vi "Serial Receive Simulation.vi"() -> ()   [LabVIEW 2013]
uses:
  <vilib>/rvi/DesktopExecutionNode/Execution/niFpgaDEN_Execute.vi
  <vilib>/rvi/DesktopExecutionNode/DesktopExecutionNode.xnode
  Source/I2S-TDM.lvlib
panel:
  out "number":u32
  out "sample bits":bool[](array[boolean])=[TRUE, FALSE, FALSE, FALSE, FALSE, FALSE, FALSE, FALSE, FALSE, FALSE, FALSE, FALSE, FALSE, FALSE, FALSE, FALSE, FALSE, FALSE, FALSE, FALSE, FALSE, FALSE, FALSE, TRUE]
  out "sample":u32
  in  "force stop":bool
  in  "start transfer":bool
  in  "ready for output":bool
  in  "pause":bool
  in  "24-bit data":bool[](array[boolean])=[TRUE, FALSE, FALSE, FALSE, FALSE, FALSE, FALSE, FALSE, FALSE, FALSE, FALSE, FALSE, FALSE, FALSE, FALSE, FALSE, FALSE, FALSE, FALSE, FALSE, FALSE, FALSE, FALSE, TRUE]
  in  "History Size":i32=100
  in  "Reset?":bool
  in  "wait":u32=50
  out "Digital Waveform Graph":digitalwaveform(graph)
  in  "transfer length":u8=32
  in  "stop":bool
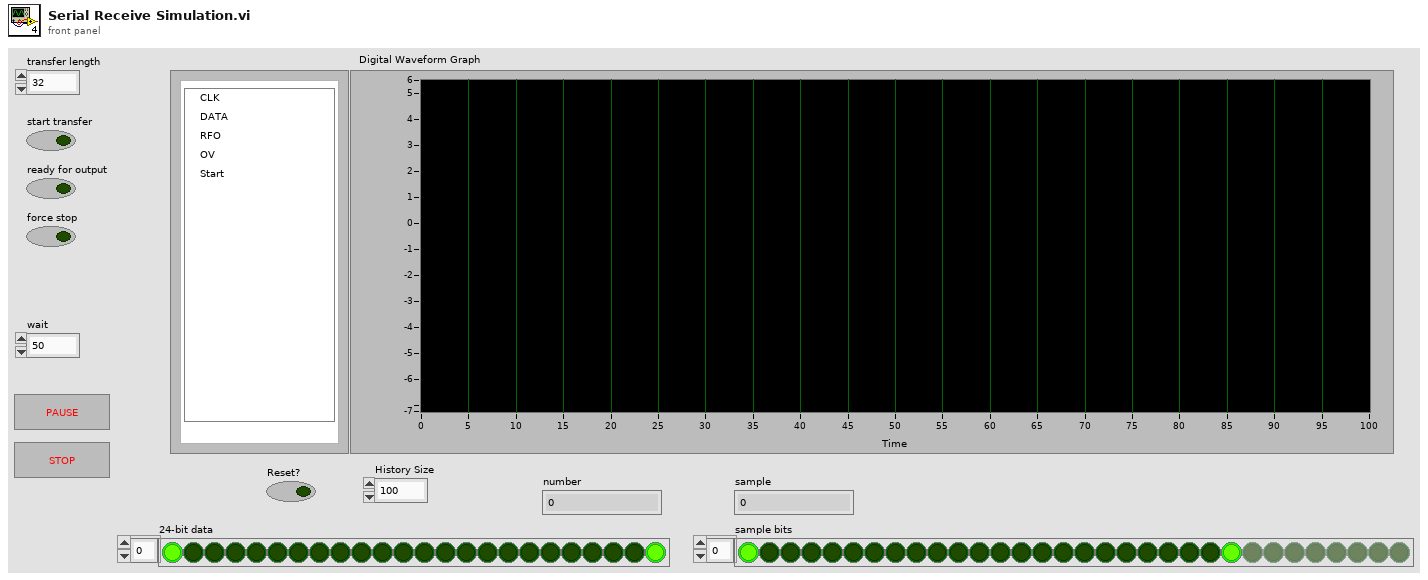
[diagram p1: front panel]
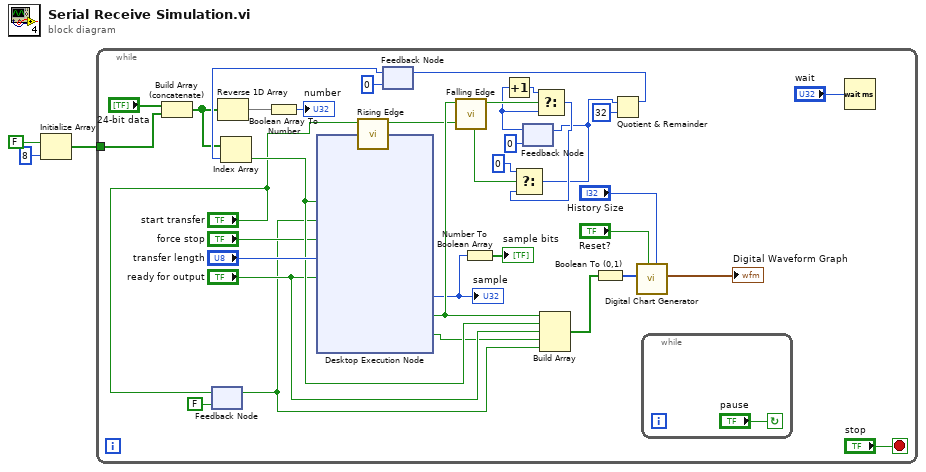
[diagram p0: block diagram]
diagram:
  n1 = Initialize Array(FALSE, 8 ("dimension size")) -> (w1:bool[])
  n2 = while {
    tunnel: w1 -> [w32]
    stop <- "stop" stop-if-true
    n3 = Build Array (concatenate)("24-bit data", w32) -> (w8:bool[])
    n4 = feedback-in #1("start transfer") -> ()
    n5 = feedback #1(FALSE ("start transfer")) -> (w6:bool)
    n6 = Reverse 1D Array(array=w8) -> (reversed array=w4:bool[])
    n7 = Boolean Array To Number(Boolean array=w4) -> (number=→"number":u32)
    n8 = call "Rising Edge.vi"("signal in"="start transfer") -> ("rising edge?"=w13:bool)  [unwired: 10 in]
    n9 = feedback #2(0) -> (w21:i32)
    n10 = Index Array(array=w8, index=w21) -> (element=w19:bool)
    n11 = xnode "Desktop Execution Node"("sdata"=w19, "start transfer"=w6, "force stop"="force stop", "transfer length"="transfer length", "ready for output"="ready for output") -> ("sample"=w15:u32, "clk"=w29:bool, "output valid"=w17:bool)  [unwired: 1 in, 1 out]
    "sample" <- w15
    n12 = call "Falling Edge.vi"("signal in"=w29) -> ("falling edge?"=w28:bool)  [unwired: 10 in]
    n13 = Number To Boolean Array(number=w15) -> (Boolean array=→"sample bits":bool[])
    n14 = feedback #3(0) -> (w26:i32)
    n15 = Increment(x=w26) -> (x+1=w25:i32)
    n16 = Select(t=w25, s=w28, f=w26) -> (s? t:f=w11:i32)
    n17 = Select(t=0, s=w13, f=w11) -> (s? t:f=w10:i32)
    n18 = feedback-in #3(w10) -> ()
    n19 = Build Array(w29, w19, "ready for output", w17, w6) -> (w30:bool[])
    n20 = Boolean To (0,1)(Boolean=w30) -> (0, 1=w31:i16[])
    n21 = Quotient & Remainder(x=w10, y=32) -> (x-y*floor(x/y)=w23:i32)  [unwired: 1 out]
    n22 = feedback-in #2(w23) -> ()
    n23 = call "Digital Chart Generator.vi"("History Size"="History Size", "Reset?"="Reset?", "Input"=w31) -> ("Digital Data"=→"Digital Waveform Graph":digitalwaveform)  [unwired: 8 in]
    n24 = while {
      stop <- "pause" continue-if-true
    }
    n25 = Wait (ms)(milliseconds to wait="wait") -> ()  [unwired: 1 out]
  }
